vi "Boolean to JSON Value.vi"(1 "Value":bool, 2 "Name":string="hello") -> (0 "JSON Value":string)   [LabVIEW 2011, in "LV JSON.lvlib"]
uses:
  LV JSON.lvlib
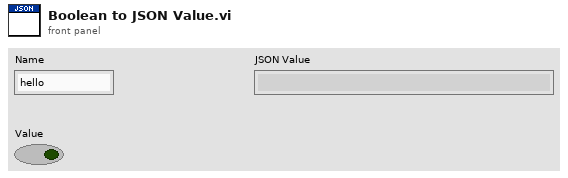
[diagram p1: front panel]
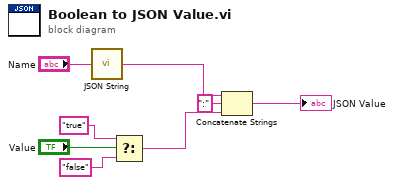
[diagram p0: block diagram]
diagram:
  n1 = call "JSON String.vi"("in"="Name") -> ("out"=w7:string)
  n2 = Select(t="true", s="Value", f="false") -> (s? t:f=w2:string)
  n3 = Concatenate Strings(w7, ":" ("string"), w2) -> (→"JSON Value":string)
